vi "Render to Writer.vi"(7 "Data":refnum<class "Abstract.lvclass">, 8 "Error In":errorcluster, 10 "Writer In":refnum<class "Abstract.lvclass">, 11 "Template":refnum<class "Template.lvclass">) -> (0 "Error Out":errorcluster, 3 "Writer Out":refnum<class "Abstract.lvclass">)   [LabVIEW 2018, in "Toolkit.lvlib"]
uses:
  Toolkit.lvlib
  Writers/Abstract/Abstract.lvclass
  Data/Abstract/Abstract.lvclass
  Nodes/Root/Template.lvclass
  Nodes/Abstract/Abstract.lvclass
  Data/Context/Context.lvclass
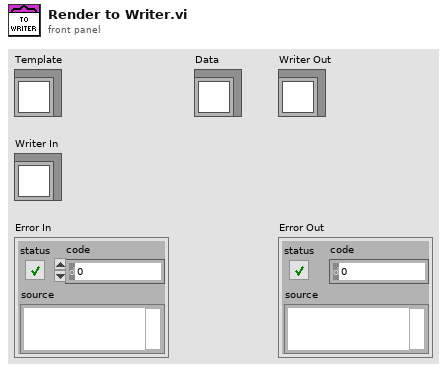
[diagram p1: front panel]
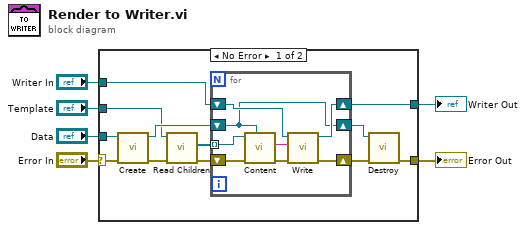
[diagram p0: block diagram]
diagram:
  n1 = case shown="No Error" "Error In" {
    selector: "Error In" -> [w16 w27]
    tunnel: [w7 w27] -> w5
    tunnel: "Writer In" -> [w18 _]
    tunnel: [w17 _] -> w3
    tunnel: "Data" -> [w14 _]
    tunnel: "Template" -> [w12 _]
    frame No Error {
      n2 = call "Create.vi"("Error In"=w16, "Data"=w14) -> ("Error Out"=w15:errorcluster, "Context"=w13:refnum<class "Context.lvclass">)  [unwired: 8 in]
      n3 = call-dynamic "Read Children.vi"("Error In"=w15, "NonTerminal In"=w12) -> ("Error Out"=w10:errorcluster, "Children"=w11:refnum<class "Abstract.lvclass">[])  [unwired: 7 in, 1 out]
      n4 = for {
        tunnel: w11 -> [w22] mode=indexing
        shift-right: [w23] -> w8
        shift-left: w10 -> [w26]
        shift-right: [w24] -> w17
        shift-left: w18 -> [w25]
        shift-right: [w19] -> w9
        shift-left: w13 -> [w19]
        n5 = call-dynamic "Content.vi"("Context"=w19, "Error In"=w26, "Abstract In"=w22) -> ("Error Out"=w20:errorcluster, "Content"=w21:string)  [unwired: 6 in, 1 out]
        n6 = call-dynamic "Write.vi"("Error In"=w20, "Content"=w21, "Writer In"=w25) -> ("Error Out"=w23:errorcluster, "Writer Out"=w24:refnum<class "Abstract.lvclass">)  [unwired: 7 in]
      }
      n7 = call "Destroy.vi"("Error In"=w8, "Context"=w9) -> ("Error Out"=w7:errorcluster)  [unwired: 9 in]
    }
    frame Error {
    }
  }
  "Error Out" <- w5
  "Writer Out" <- w3
